vi "SCMP - Error Handling - Verify All Recipes Exist.vi"(8 "error in (no error)":errorcluster, 11 "List of Recipes":path[](array[path])=[path "c:/PDSS_observer_cbks_rcps/recipes/6563\t6563.rcp", path "c:/PDSS_observer_cbks_rcps/recipes/8542\t8542.rcp", path "c:/PDSS_observer_cbks_rcps/recipes/10830\t10830.rcp"]) -> (0 "error out":errorcluster, 1 "Recipe Not Found":path, 2 "max Cookbook Exposure [ms]":i32, 3 "min Cookbook Exposure [ms]":i32)   [LabVIEW 2014]
doc: "Use this template to build a VI to use as a subVI."
panel:
  out "# of recepies":i32
  out "Recipe Not Found":bool[](array[boolean])=[TRUE, TRUE, TRUE]
  out "All paths good":bool=TRUE
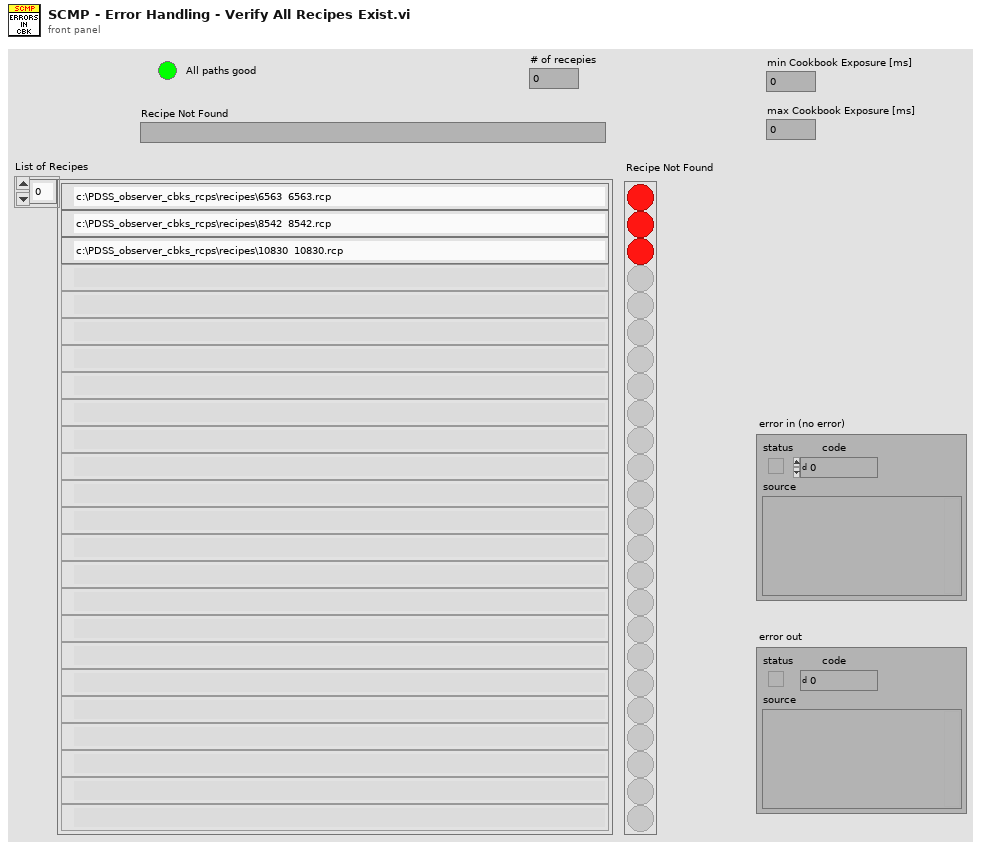
[diagram p1: front panel]
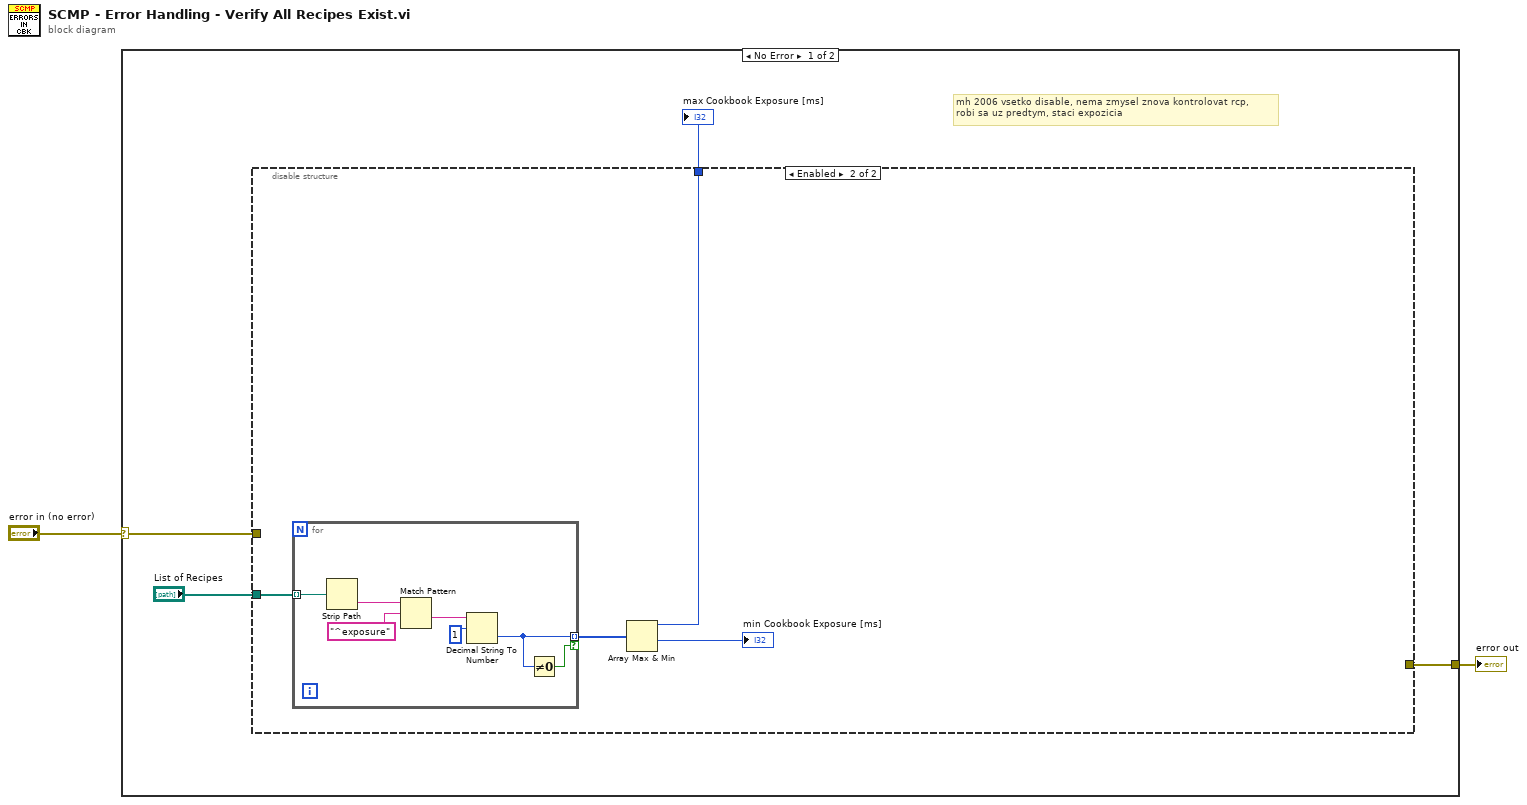
[diagram p0: block diagram]
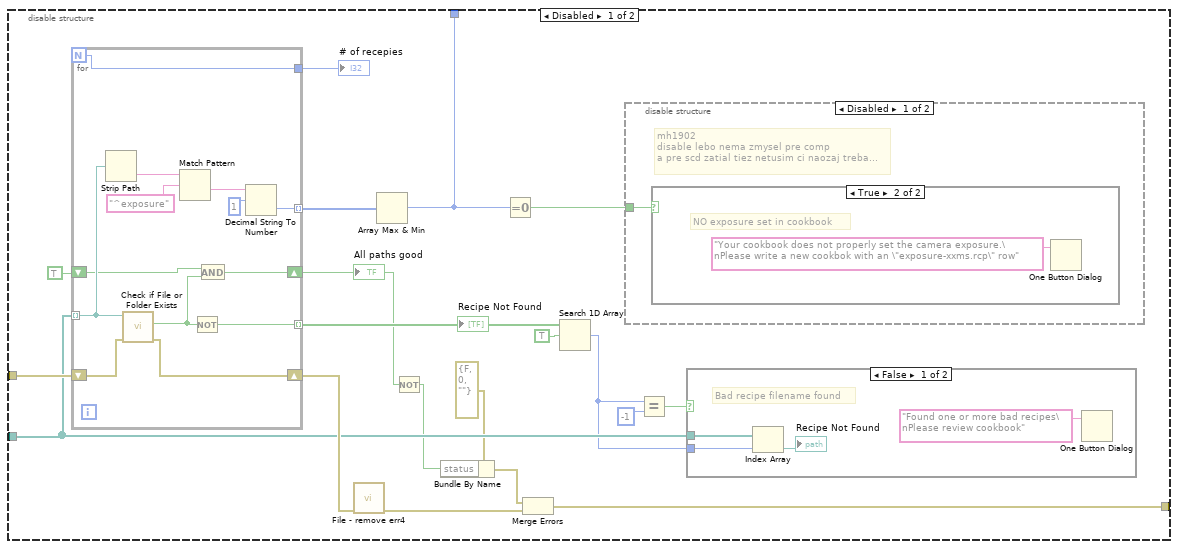
[diagram p2: hidden frame]
diagram:
  n1 = case shown="No Error" "error in (no error)" {
    selector: "error in (no error)" -> [w6 w56]
    tunnel: [w4 w56] -> w1
    frame No Error {
      # "mh 2006 vsetko disable, nema zmysel znova kontrolovat rcp, \nrobi sa uz predtym, staci expozicia"
      n2 = disable-structure shown="Enabled" {
        disable-tunnel: w6 -> [w25 _]
        disable-tunnel: "List of Recipes" -> [w16 w47]
        disable-tunnel: [w12 _] -> w4
        disable-tunnel: [w7 w46] -> w3
        frame Disabled {
          n3 = for {
            N -> [w35]
            tunnel: w16 -> [w41] mode=indexing
            shift-right: [w43] -> w22
            shift-left: w25 -> [w44]
            shift-right: [w34] -> w8
            shift-left: TRUE ("file or folder exists?") -> [w32]
            tunnel: [w42] -> w20 mode=indexing
            tunnel: [w37] -> w14 mode=indexing
            tunnel: [w35] -> w15
            n4 = Strip Path(path=w41) -> (name=w40:string)  [unwired: 1 out]
            n5 = call <vilib>:"Check if File or Folder Exists.vi"("error in (no error)"=w44, "path"=w41) -> ("error out"=w43:errorcluster, "file or folder exists?"=w33:bool)  [unwired: 7 in, 1 out]
            n6 = Match Pattern(string=w40, regular expression="^exposure") -> (after substring=w38:string)  [unwired: 1 in, 3 out]
            n7 = Not(x=w33) -> (.not. x?=w42:bool)
            n8 = And(x=w32, y=w33) -> (x .and. y?=w34:bool)
            n9 = Decimal String To Number(string=w38, offset=1) -> (number=w37:i32)  [unwired: 1 in, 1 out]
          }
          "All paths good" <- w8
          "Recipe Not Found" <- w20
          "# of recepies" <- w15
          n10 = call "File - remove err4.vi"("error in (no error)"=w22) -> ("error out"=w23:errorcluster)  [unwired: 10 in]
          n11 = Array Max & Min(array=w14) -> (max value=w7:i32)  [unwired: 3 out]
          n12 = Not(x=w8) -> (.not. x?=w9:bool)
          n13 = Bundle By Name(cluster=errorcluster {"status"=FALSE, "code"=0, "source"=""} ("error in"), "status"=w9) -> (w10:errorcluster)
          n14 = Equal To 0?(x=w7) -> (x = 0?=w21:bool)
          n15 = Merge Errors(w10, w23) -> (w12:errorcluster)
          n16 = Search 1D Array(1D array=w20, element=TRUE) -> (index of element=w13:i32)  [unwired: 1 in]
          n17 = disable-structure shown="Disabled" {
            disable-tunnel: w21 -> [w26 _]
            frame Disabled {
              # "mh1902 \ndisable lebo nema zmysel pre comp\na pre scd zatial tiez netusim ci naozaj treba..."
              n18 = case shown="True" w26 {
                frame False {
                }
                frame True {
                  # "NO exposure set in cookbook"
                  n19 = One Button Dialog(message="Your cookbook does not properly set the camera exposure.\nPlease write a new cookbok with an \"exposure-xxms.rcp\" row") -> ()  [unwired: 1 in, 1 out]
                }
              }
            }
            frame Enabled {
            }
          }
          n20 = Equal?(x=w13, y=-1) -> (x = y?=w17:bool)
          n21 = case shown="False" w17 {
            tunnel: w16 -> [w30 _]
            tunnel: w13 -> [w29 _]
            frame False {
              # "Bad recipe filename found"
              n22 = Index Array(array=w30, index=w29) -> (element=→"Recipe Not Found":path)
              n23 = One Button Dialog(message="Found one or more bad recipes\nPlease review cookbook") -> ()  [unwired: 1 in, 1 out]
            }
            frame True {
              # "All recipes are good"
            }
          }
        }
        frame Enabled {
          n24 = for {
            tunnel: [w49] -> w48 mode=indexing if=w50
            tunnel: w47 -> [w51] mode=indexing
            n25 = Strip Path(path=w51) -> (name=w55:string)  [unwired: 1 out]
            n26 = Match Pattern(string=w55, regular expression="^exposure") -> (after substring=w53:string)  [unwired: 1 in, 3 out]
            n27 = Decimal String To Number(string=w53, offset=1) -> (number=w49:i32)  [unwired: 1 in, 1 out]
            n28 = Not Equal To 0?(x=w49) -> (x != 0?=w50:bool)
          }
          n29 = Array Max & Min(array=w48) -> (max value=w46:i32, min value=→"min Cookbook Exposure [ms]":i32)  [unwired: 2 out]
        }
      }
      "max Cookbook Exposure [ms]" <- w3
    }
    frame Error {
    }
  }
  "error out" <- w1
